vi "Assert Greater Or Equal_Variant.vi"(4 "Execution time (s)":dbl=-1.0, 5 "Assert Only? (F)":bool, 6 "error code (1)":i32=1, 7 "Label":string, 8 "error in (no error)":errorcluster, 10 "Y":variant, 11 "X":variant) -> (0 "error out":errorcluster)   [LabVIEW 2013, in "Caraya.lvlib" / "Assert.lvclass"]
doc: "Generates an error if the input condition is not met.\n\n--\nCopyright © 2015 JKI All rights reserved.\n\nAuthor: Tomi Maila <tomi.maila@jki.net>\n\nThis library is provided \"AS IS\" ,WITHOUT WARRANTIES OR\nCONDITIONS OF ANY KIND, either express or implied.\n\nJKI -- jki.net"
uses:
  Assert.lvclass
panel:
  # "Copyright © 2015 JKI All rights reserved.\n\nAuthor: Tomi Maila <tomi.maila@jki.net>\n\nThis library is provided \"AS IS\" ,WITHOUT WARRANTIES OR\nCONDITIONS OF ANY KIND, either express or implied.\n\nJKI -- jki.net"
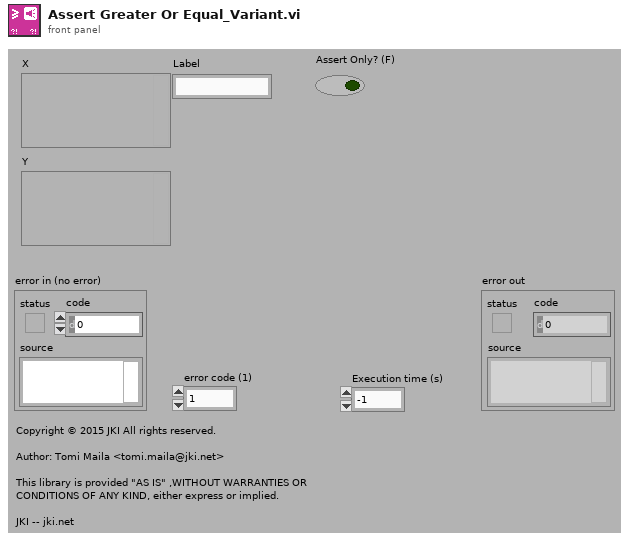
[diagram p1: front panel]
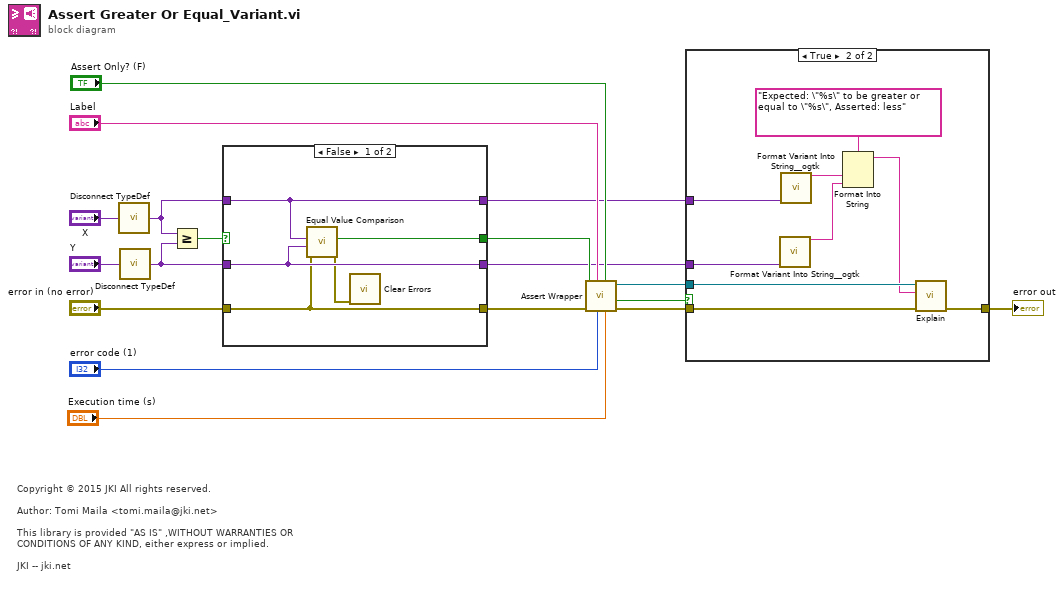
[diagram p0: block diagram]
diagram:
  # "Copyright © 2015 JKI All rights reserved.\n\nAuthor: Tomi Maila <tomi.maila@jki.net>\n\nThis library is provided \"AS IS\" ,WITHOUT WARRANTIES OR\nCONDITIONS OF ANY KIND, either express or implied.\n\nJKI -- jki.net"
  n1 = call "Disconnect TypeDef.vi"("Variant"="X") -> ("Variant Out"=w8:variant)
  n2 = call "Disconnect TypeDef.vi"("Variant"="Y") -> ("Variant Out"=w4:variant)
  n3 = Greater Or Equal?(x=w8, y=w4) -> (x >= y?=w6:bool)
  n4 = case shown="False" w6 {
    selector: w6 -> [_ w26]
    tunnel: w8 -> [w23 w27]
    tunnel: [w23 w27] -> w7
    tunnel: [w21 w26] -> w5
    tunnel: w4 -> [w22 w25]
    tunnel: [w22 w25] -> w3
    tunnel: "error in (no error)" -> [w20 w24]
    tunnel: [w20 w24] -> w1
    frame False {
      n5 = call "Equal Value Comparison.vi"("error in (no error)"=w20, "Y"=w22, "X"=w23) -> ("error out"=w19:errorcluster, "Equal Values?"=w21:bool)  [unwired: 6 in, 1 out]
      n6 = call <vilib>:"Clear Errors.vi"("error in (no error)"=w19) -> ()  [unwired: 6 in, 1 out]
    }
    frame True {
    }
  }
  n7 = call "Assert Wrapper.vi"("Execution time (s)"="Execution time (s)", "Assert Only? (F)"="Assert Only? (F)", "error code (1)"="error code (1)", "Label"="Label", "error in (no error)"=w1, "Assert?"=w5) -> ("error out"=w14:errorcluster, "Verbose"=w11:bool, "Assert out"=w12:refnum<class "Assert.lvclass">)  [unwired: 3 in]
  n8 = case shown="True" w11 {
    tunnel: [w28 w37] -> w13
    tunnel: w12 -> [_ w36]
    tunnel: w14 -> [w28 w35]
    tunnel: w7 -> [_ w33]
    tunnel: w3 -> [_ w29]
    frame False {
    }
    frame True {
      n9 = call <userlib>:"Format Variant Into String__ogtk.vi"("Variant"=w29) -> ("Output String"=w30:string)  [unwired: 13 in, 1 out]
      n10 = call <userlib>:"Format Variant Into String__ogtk.vi"("Variant"=w33) -> ("Output String"=w31:string)  [unwired: 13 in, 1 out]
      n11 = Format Into String(format string="Expected: \"%s\" to be greater or equal to \"%s\", Asserted: less" ("t"), w31, w30) -> (resulting string=w34:string)  [unwired: 2 in, 1 out]
      n12 = call-dynamic "Explain.vi"("error in (no error)"=w35, "Verbose Explanation"=w34, "Assert in"=w36) -> ("error out"=w37:errorcluster)  [unwired: 7 in, 1 out]
    }
  }
  "error out" <- w13
